vi "formula.vi"() -> ()   [LabVIEW 2015]
panel:
  out "Waveform Graph":dbl[](graph)
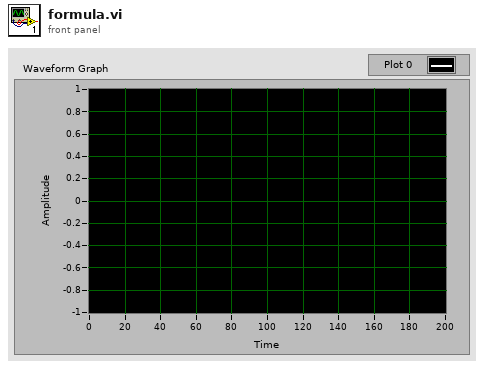
[diagram p1: front panel]
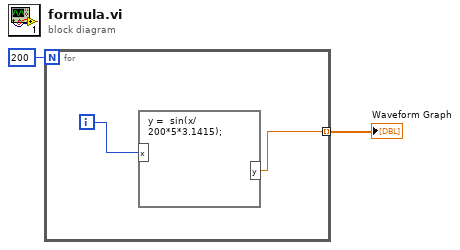
[diagram p0: block diagram]
diagram:
  n1 = for {
    N: 200 -> [_]
    tunnel: [w4] -> w1 mode=indexing
    i -> [w3]
    n2 = formula code="y =  sin(x/200*5*3.1415);"("x"=w3) -> ("y"=w4:dbl)
  }
  "Waveform Graph" <- w1
